vi "Get PID Values.vi"(8 "error in (no error)":errorcluster, 11 "Modbus Master in":refnum<class "Modbus Master.lvclass">) -> (0 "error out":errorcluster, 2 "register values":dbl[](array[numeric]), 3 "Modbus Master out":refnum<class "Modbus Master.lvclass">)   [LabVIEW 2023, in "PIDModbus.lvlib"]
uses:
  PIDModbus.lvlib
  <vilib>/NI/Modbus Library/API/Master/Modbus Master.lvclass
  Controls/Register Enum.ctl
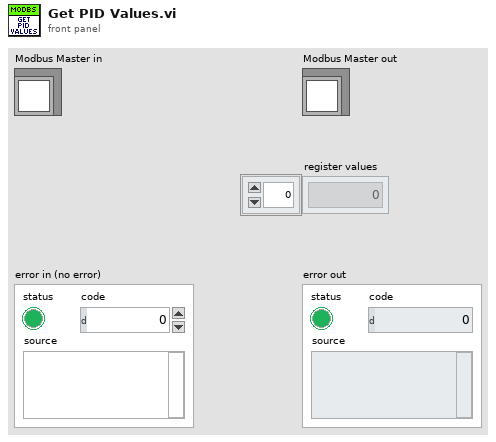
[diagram p1: front panel]
types:
  T1 = typedef "PIDModbus.lvlib/Register Enum.ctl" = u16
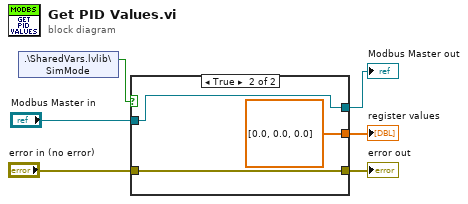
[diagram p0: block diagram]
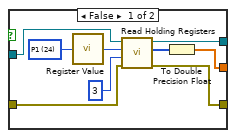
[diagram p2: hidden frame]
diagram:
  n1 = shared-variable ".\\SharedVars.lvlib\\SimMode"() -> (w1:bool)  [unwired: 1 in, 1 out]
  n2 = case shown="True" w1 {
    tunnel: [w15 w17] -> w6
    tunnel: [w14 w18] -> w5
    tunnel: "error in (no error)" -> [w11 w17]
    tunnel: "Modbus Master in" -> [w10 w18]
    tunnel: [w7 dbl[] [0.0, 0.0, 0.0]] -> w2
    frame False {
      w9 = T1 24 items=["PV"=0, "SV"=5, "P1"=24, "I1"=25, "D1"=26] ("Register")
      n3 = call "Register Value.vi"("Register"=w9) -> ("RegAddr (Hex)"=w8:u16)
      n4 = call-dynamic "Read Holding Registers.vi"("error in"=w11, "number of inputs"=u16 3, "starting address"=w8, "Modbus master in"=w10) -> ("error out"=w15:errorcluster, "register values"=w13:u16[], "Modbus master out"=w14:refnum<class "Modbus Master.lvclass">)  [unwired: 5 in]
      n5 = To Double Precision Float(number=w13) -> (double precision float=w7:dbl[])
    }
    frame True {
    }
  }
  "error out" <- w6
  "Modbus Master out" <- w5
  "register values" <- w2
